vi "Facade.vi"(0 "Data In":T4, 2 "Display State In":T2, 3 "Container State":T3) -> (6 "Data Out":T4, 7 "Display State Out":T2, 8 "Action":T1)   [LabVIEW 2020, in "KMultilevel Ring.xctl"]
uses:
  KMultilevel Ring.xctl
  Data.ctl
  <vilib>/_xctls/Container State.ctl
  State.ctl
  <vilib>/_xctls/Action.ctl
  <vilib>/_xctls/XControlSupport.lvlib
panel:
  in  "Ring":u16(ring)
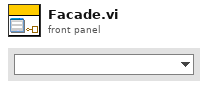
[diagram p1: front panel]
types:
  T1 = typedef "XControlSupport.lvlib/Action.ctl" = cluster{"Data Changed?":bool, "State Changed?":bool, "Action Name":string}
  T2 = typedef "KMultilevel Ring.xctl/State.ctl" = cluster{"Strings":string[], "delimiter":string}
  T3 = typedef "XControlSupport.lvlib/Container State.ctl" = cluster{"Indicator?":bool, "Run Mode?":bool, " Refnum":refnum<vi>}
  T4 = typedef "KMultilevel Ring.xctl/Data.ctl" = string
  T5 = enum8{"Enabled", "Disabled", "Disabled and Grayed Out"}
  T6 = cluster{"Names":string[], "Tags":string[], "Child":i32[]}[]
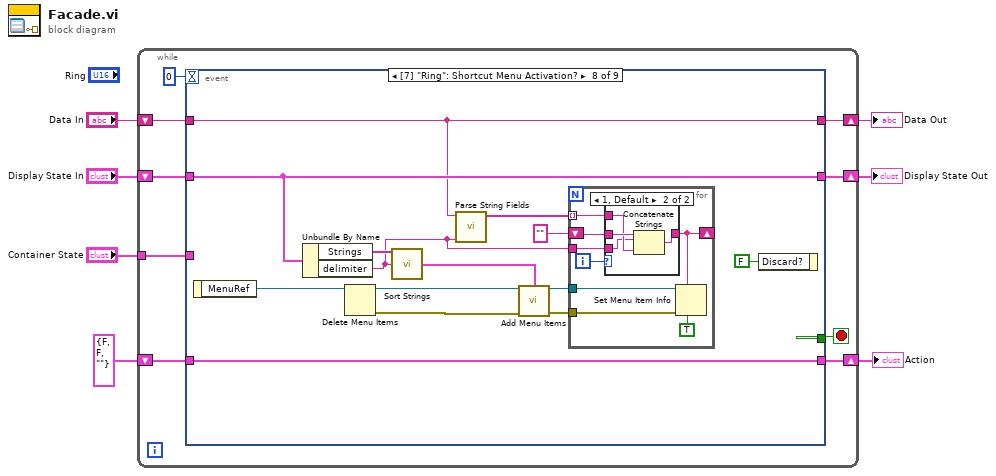
[diagram p0: block diagram]
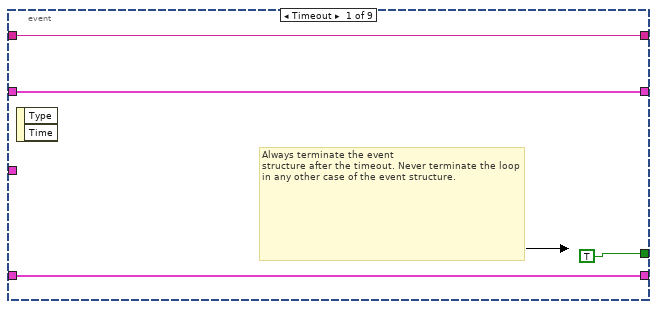
[diagram p2: hidden frame]
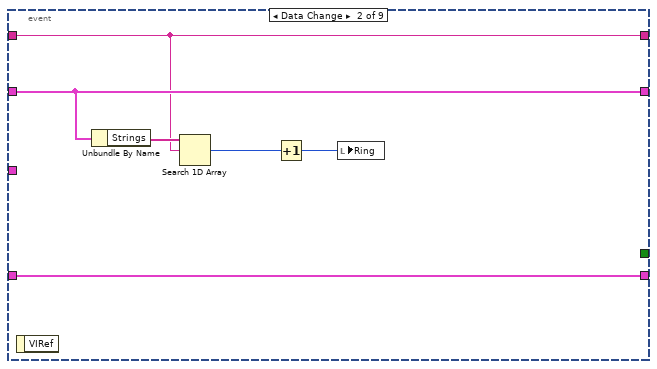
[diagram p3: hidden frame]
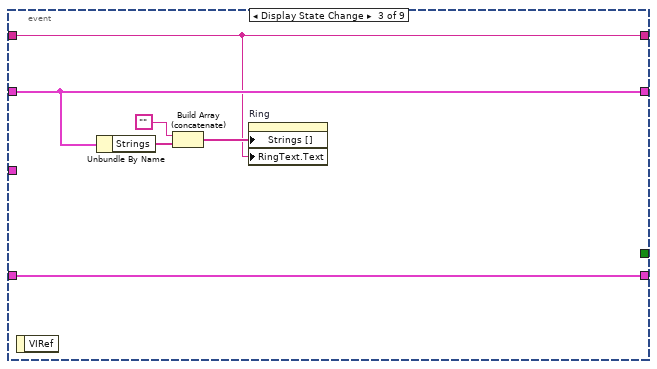
[diagram p4: hidden frame]
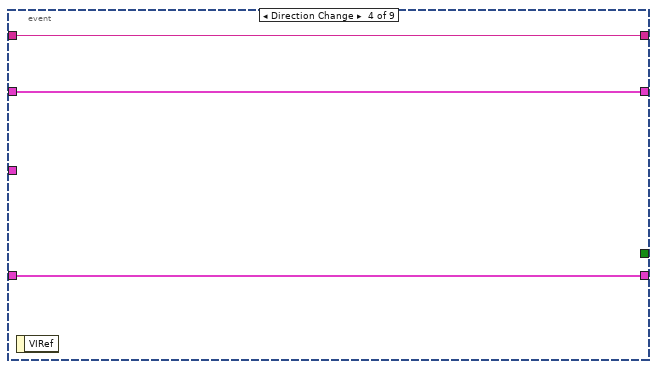
[diagram p5: hidden frame]
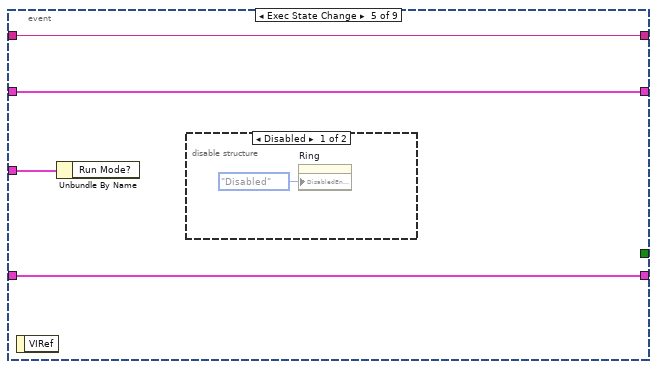
[diagram p6: hidden frame]
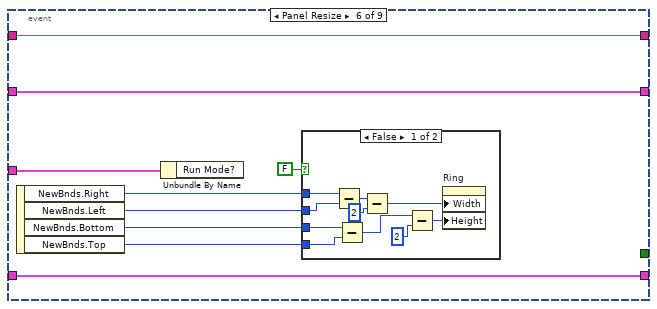
[diagram p8: hidden frame]
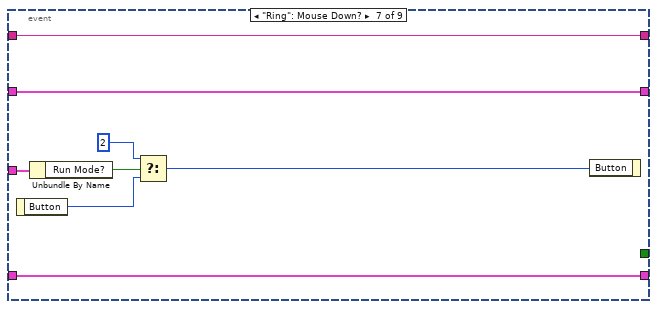
[diagram p10: hidden frame]
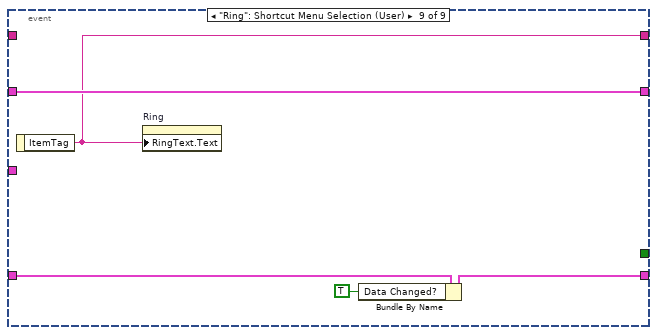
[diagram p12: hidden frame]
diagram:
  n1 = while {
    shift-right: [w15] -> w4
    shift-left: "Display State In" -> [w16]
    tunnel: "Container State" -> [w12]
    shift-right: [w10] -> w7
    shift-left: "Data In" -> [w11]
    shift-right: [w8] -> w2
    shift-left: T1 {"Data Changed?"=FALSE, "State Changed?"=FALSE, "Action Name"=""} ("Action") -> [w9]
    stop <- w14 stop-if-true
    n2 = event shown="[7] \"Ring\": Shortcut Menu Activation?" {
      selector: _ -> [_ _ _ _ _ _ _ _ _]
      dyn-events: _ -> [_ _ _ _ _ _ _ _ _]
      timeout: 0 -> [_ _ _ _ _ _ _ _ _]
      tunnel: w16 -> [w18 w25 w31 w35 w38 w49 w67 w80 w99]
      tunnel: [w18 w25 w31 w35 w38 w49 w67 w80 w99] -> w15
      tunnel: [TRUE _ _ _ _ _ _ _ _] -> w14
      tunnel: w12 -> [_ _ _ _ w39 w46 w64 _ _]
      tunnel: w11 -> [w17 w23 w27 w34 w37 w48 w66 w68 _]
      tunnel: [w17 w23 w27 w34 w37 w48 w66 w68 w97] -> w10
      tunnel: [w19 w26 w32 w33 w36 w47 w65 w81 w96] -> w8
      tunnel: w9 -> [w19 w26 w32 w33 w36 w47 w65 w81 w98]
      event Timeout {
        # "Always terminate the event\nstructure after the timeout. Never terminate the loop in any other case of the event structure."
        n3 = event-data() -> ()  [unwired: 1 in, 2 out]
      }
      event Data Change {
        n4 = event-data() -> ()  [unwired: 1 in, 1 out]
        n5 = Unbundle By Name(w25) -> ("Strings"=w24:string[])
        n6 = Search 1D Array(1D array=w24, element=w23) -> (index of element=w22:i32)  [unwired: 1 in]
        n7 = Increment(x=w22) -> (x+1=w21:i32)
        n8 = local write "Ring"(w21) -> ()
      }
      event Display State Change {
        n9 = event-data() -> ()  [unwired: 1 in, 1 out]
        n10 = Unbundle By Name(w31) -> ("Strings"=w30:string[])
        n11 = Build Array (concatenate)("", w30) -> (w29:string[])
        n12 = property on="Ring" class="Ring (strict)"("Strings []"=w29, "RingText.Text"=w27) -> ()  [unwired: 2 in, 2 out]
      }
      event Direction Change {
        n13 = event-data() -> ()  [unwired: 1 in, 1 out]
      }
      event Exec State Change {
        n14 = event-data() -> ()  [unwired: 1 in, 1 out]
        n15 = Unbundle By Name(w39) -> ()  [unwired: 1 out]
        n16 = disable-structure shown="Disabled" {
          frame Disabled {
            n17 = property on="Ring" class="Ring (strict)"("DisabledEnum"=T5."Disabled" ("Disabled")) -> ()  [unwired: 2 in, 2 out]
          }
          frame Enabled {
          }
        }
      }
      event Panel Resize {
        n18 = event-data() -> ("NewBnds.Right"=w45:i16, "NewBnds.Left"=w44:i16, "NewBnds.Bottom"=w43:i16, "NewBnds.Top"=w42:i16)  [unwired: 1 in]
        n19 = Unbundle By Name(w46) -> ()  [unwired: 1 out]
        n20 = case shown="False" FALSE {
          tunnel: w44 -> [w59 _]
          tunnel: w45 -> [w58 _]
          tunnel: w42 -> [w57 _]
          tunnel: w43 -> [w56 _]
          frame False {
            n21 = Subtract(x=w58, y=w59) -> (x-y=w55:i16)
            n22 = Subtract(x=w56, y=w57) -> (x-y=w54:i16)
            n23 = Subtract(x=w55, y=i16 2) -> (x-y=w53:i16)
            n24 = Subtract(x=w54, y=i16 2) -> (x-y=w51:i16)
            n25 = property on="Ring" class="Ring (strict)"("Width"=w53, "Height"=w51) -> ()  [unwired: 2 in, 2 out]
          }
          frame True {
          }
        }
      }
      event "Ring": Mouse Down? {
        n26 = event-data() -> ("Button"=w62:u16)  [unwired: 1 in]
        n27 = Unbundle By Name(w64) -> ("Run Mode?"=w63:bool)
        n28 = Select(t=u16 2, s=w63, f=w62) -> (s? t:f=w60:u16)
        n29 = event-data("Button"=w60) -> ()  [unwired: 1 in, 1 out]
      }
      event "Ring": Shortcut Menu Activation? {
        n30 = event-data() -> ("MenuRef"=w78:refnum<k9>)  [unwired: 1 in]
        n31 = Unbundle By Name(w80) -> ("Strings"=w77:string[], "delimiter"=w69:string)
        n32 = Delete Menu Items(9:w78) -> (0:w75:errorcluster, 3:w76:refnum<k9>)  [unwired: 3 in]
        n33 = call "Sort Strings.vi"("Strings"=w77, "Delimiter"=w69) -> ("Menu Items"=w74:T6)  [unwired: 13 in]
        n34 = call "Parse String Fields.vi"("Separator"=w69, "String"=w68) -> ("Fields"=w71:string[])  [unwired: 8 in, 1 out]
        n35 = call "Add Menu Items.vi"("Menu in"=w76, "Menu Items"=w74, "error in (no error)"=w75) -> ("Menu out"=w72:refnum<k9>, "error out"=w73:errorcluster)  [unwired: 11 in]
        n36 = for {
          tunnel: w73 -> [w89]
          tunnel: w72 -> [w88]
          tunnel: w71 -> [w84] mode=indexing
          shift-right: [w85] -> _
          shift-left: "" -> [w86]
          tunnel: w69 -> [w82]
          i -> [w83]
          n37 = case shown="1, Default" w83 {
            tunnel: w86 -> [_ w94]
            tunnel: [w90 w93] -> w85
            tunnel: w84 -> [w90 w92]
            tunnel: w82 -> [_ w91]
            frame 0 {
            }
            frame 1, Default {
              n38 = Concatenate Strings(w94, w91, w92) -> (w93:string)
            }
          }
          n39 = Set Menu Item Info(6:TRUE ("checked"), 7:w85, 8:w89, 11:w88) -> ()  [unwired: 3 in, 2 out]
        }
        n40 = event-data("Discard?"=FALSE) -> ()  [unwired: 1 in, 1 out]
      }
      event "Ring": Shortcut Menu Selection (User) {
        n41 = event-data() -> ("ItemTag"=w97:string)  [unwired: 1 in]
        n42 = property on="Ring" class="Ring (strict)"("RingText.Text"=w97) -> ()  [unwired: 2 in, 2 out]
        n43 = Bundle By Name(cluster=w98, "Data Changed?"=TRUE) -> (w96:T1)
      }
    }
  }
  "Display State Out" <- w4
  "Data Out" <- w7
  "Action" <- w2
